vi "Subvi AO LUT mon.vi"(1 "AO mon":refnum<k21>="Connector1/AO1", 2 "AO":refnum<k21>="Connector1/AO0", 7 "Ext trig enable":bool, 9 "FIFO In":refnum<k21>="GALVO1mem") -> ()   [LabVIEW 2017]
uses:
  <vilib>/Platform/TimedLoop/XDataNode/timing_clust.ctl
  <vilib>/Platform/TimedLoop/XDataNode/nitl_modes.ctl
  <vilib>/Platform/TimedLoop/XDataNode/wakeup.ctl
  <vilib>/rvi/Emulation/niFpgaSctlEmulationGetInTimedLoop.vi
  <vilib>/rvi/Emulation/niFpgaEmulationReportErrorSimple.vi
  <vilib>/rvi/Emulation/niFpgaGetClockAttributes.vi
  <vilib>/rvi/Emulation/niFpgaCriticalErrorInLSC.vi
  Detector/GV gated frameclock.vi
  Detector/GV framegate.vi
  <vilib>/rvi/DataTransferAndStorage/Container/Common/niFpgaContainerExecOnDevCompGetState.vi
  <vilib>/rvi/Emulation/niFpgaEmulationIsFPGAContextNoSignature.vi
  <vilib>/rvi/DataTransferAndStorage/Container/Common/niFpgaContainerGetUniqueNameForEmu.vi
  <vilib>/rvi/Emulation/niFpgaProcessEmulError.vi
  <vilib>/rvi/errors/nirviReportUnexpectedCaseInternalError (U32).vi
  <vilib>/rvi/Memory/Memory_Emulation/niFpgaMemoryEmulationCacheClearOnFirstRun.vi
  <vilib>/rvi/Memory/Memory_Emulation/nirvimemoryEmulationManagerCache_MakeExclusive.vi
  <vilib>/rvi/Memory/Memory_Emulation/niFpgaMemoryEmulationValidateCache.vi
  <vilib>/rvi/Memory/Memory_Emulation/nirvimemoryEmulationManagerCache_InsertValue.vi
  <vilib>/Utility/error.llb/Clear Errors.vi
  <vilib>/rvi/Memory/Memory_Emulation/nirvimemoryEmulationManagerCache_ReleaseExclusive.vi
  <vilib>/rvi/Memory/Memory_Emulation/nirvimemoryEmulationManagerCache_GetValue.vi
  <vilib>/rvi/Memory/Memory_Emulation/nirvimemoryEmulationManagerCache_SetValue.vi
  <vilib>/rvi/Emulation/niFpgaSctlEmulationResourceMgr.vi
  <vilib>/rvi/eio/common/nirviEmuTemplateMethod_errors.vi
  <vilib>/Platform/TimedLoop/XDataNode/XDataNode.xnode
  <vilib>/rvi/DataTransferAndStorage/Container/XNode/niFpgaContainer.xnode
  <vilib>/rvi/Memory/Memory_Emulation/niFpgaMemoryEmulationRefIn.vi
  <vilib>/eio/EIONode/EIONode.xnode
  <vilib>/Platform/TimedLoop/XDataNode/XDNodeRunTimeDep.lvlib
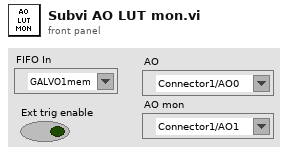
[diagram p1: front panel]
types:
  T1 = typedef "XDNodeRunTimeDep.lvlib/timing_clust.ctl" = cluster{"Expected End [f-1]":u64, "Actual End [f-1]":u64, "Finished Late? [f-1]":bool, "Expected End [i-1]":u64, "Actual End [i-1]":u64, "Finished Late? [i-1]":bool, "Expected Start [i]":u64, "Actual Start [i]":u64, "Expected Start [f]":u64, "Actual Start [f]":u64, "Source Name":string, "Structure Name":string, "Period":i64, "Deadline":i64, "Offset":i64, "Start":i64, "Priority":i32, "Timeout":i32, "Mode":T2, "Wakeup Reason":T3, "Error":errorcluster, "Source Type":string, "Secondary Source Type":string, "Global End Time":u64, "Global Start Time":u64, "Frame Duration":u64, "Iteration Duration":u64, "Assigned CPU":i32, "I/O Scan Engine Mode":u32}
  T2 = typedef "XDNodeRunTimeDep.lvlib/nitl_modes.ctl" = enum32{"No Change", "Process missed periods, maintain original phase", "Discard missed periods, maintain original phase", "Process missed periods, ignore original phase", "Discard missed periods, ignore original phase"}
  T3 = typedef "XDNodeRunTimeDep.lvlib/wakeup.ctl" = enum32{"Normal", "Aborted", "Asynchronous wakeup", "Timing source error", "Timed loop error", "Timeout"}
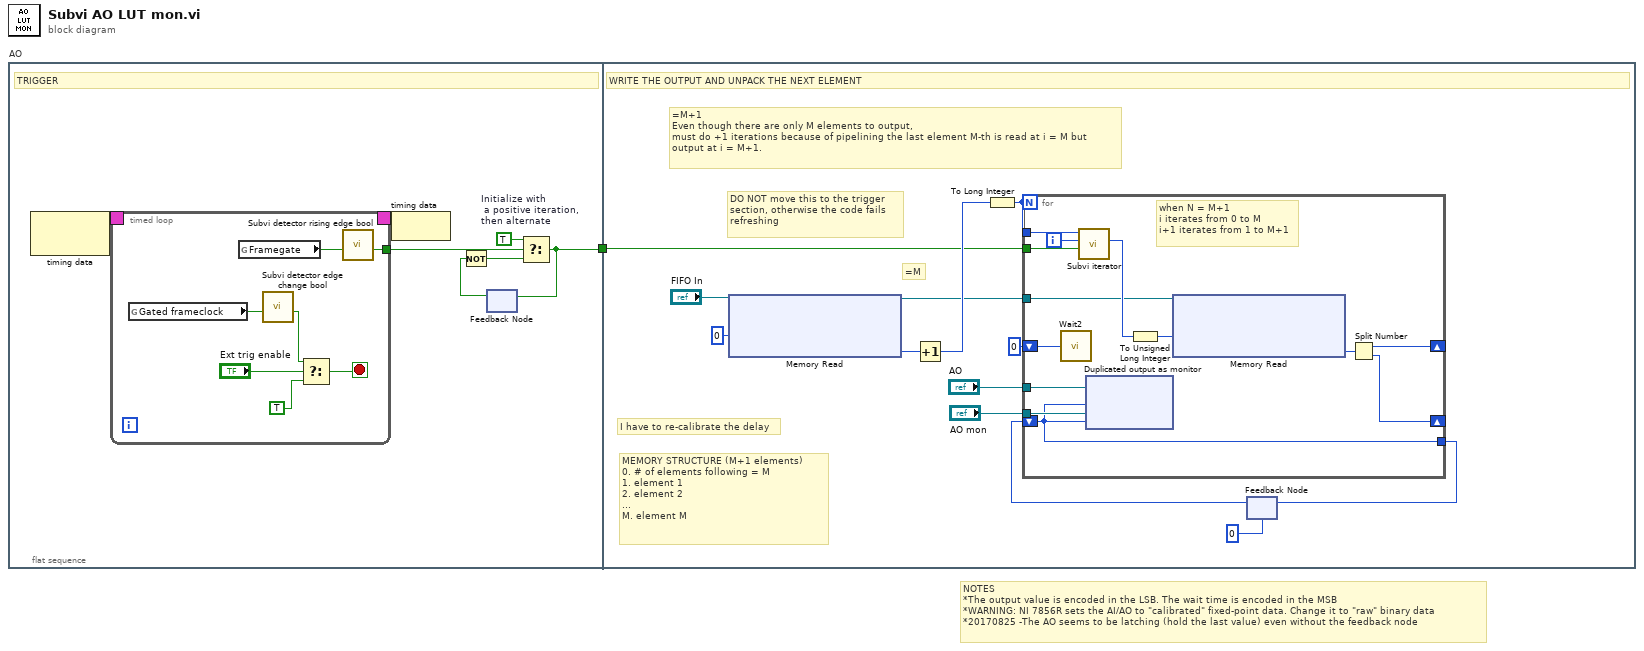
[diagram p0: block diagram]
diagram:
  # "NOTES\n*The output value is encoded in the LSB. The wait time is encoded in the MSB\n*WARNING: NI 7856R sets the AI/AO to \"calibrated\" fixed-point data. Change it to \"raw\" binary data\n*20170825 -The AO seems to be latching (hold the last value) even without the feedback node"
  n1 = flat-sequence "AO" {
    tunnel: [w2] -> w1
    tunnel: w1 -> [w24]
    frame #0 {
      # "TRIGGER"
      n2 = node-c288() -> (w8:T1)  [unwired: 1 in]
      n3 = timed-loop {
        timing: w8 -> [_]
        timing-out: [_] -> w7
        tunnel: [w9] -> w3
        stop <- w13 stop-if-true
        n4 = global read "GV gated frameclock.vi" "Gated frameclock"() -> (w12:bool)
        n5 = global read "GV framegate.vi" "Framegate"() -> (w10:bool)
        n6 = call "Subvi detector edge change bool.vi"("Input"=w12) -> ("Output"=w11:bool)  [unwired: 8 in]
        n7 = Select(t=w11, s="Ext trig enable", f=TRUE) -> (s? t:f=w13:bool)
        n8 = call "Subvi detector rising edge bool.vi"("Input"=w10) -> ("Output"=w9:bool)  [unwired: 10 in]
      }
      n9 = node-c288(w7) -> ()
      n10 = feedback #1() -> (w5:bool)  [unwired: 1 in]
      n11 = Not(x=w5) -> (.not. x?=w6:bool)
      n12 = Select "Initialize with\n a positive iteration,\nthen alternate"(t=TRUE, s=w3, f=w6) -> (s? t:f=w2:bool)
      n13 = feedback-in #1(w2) -> ()
    }
    frame #1 {
      # "DO NOT move this to the trigger\nsection, otherwise the code fails\nrefreshing"
      # "I have to re-calibrate the delay"
      # "MEMORY STRUCTURE (M+1 elements)\n0. # of elements following = M\n1. element 1\n2. element 2\n...\nM. element M"
      # "=M+1\nEven though there are only M elements to output,\nmust do +1 iterations because of pipelining the last element M-th is read at i = M but\noutput at i = M+1."
      # "=M"
      # "WRITE THE OUTPUT AND UNPACK THE NEXT ELEMENT"
      n14 = xnode ("Memory Read")("Address"=u32 0, "Memory In"="FIFO In") -> ("Data"=w26:u32, "Memory Out"=w25:refnum<k21>)
      n15 = Increment(x=w26) -> (x+1=w29:u32)
      n16 = To Long Integer(number=w29) -> (32bit integer=w28:i32)
      n17 = feedback #2(u16 0) -> (w32:u16)
      n18 = for {
        N: w28 -> [_]
        shift-right: [w43] -> _
        shift-left: u16 0 -> [w41]
        shift-right: [w42] -> _
        shift-left: w32 -> [w33]
        tunnel: [w33] -> w30
        tunnel: w28 -> [w38]
        tunnel: w24 -> [w37]
        tunnel: w25 -> [w36]
        tunnel: "AO mon" -> [w35]
        tunnel: "AO" -> [w34]
        i -> [w39]
        # "when N = M+1\ni iterates from 0 to M\ni+1 iterates from 1 to M+1"
        n19 = call "Wait2"("Count(Ticks)"=w41) -> ()  [unwired: 1 out]
        n20 = call "Subvi iterator.vi"("Set increase"=w37, "Iterator in"=w39, "Nmax"=w38) -> ("Iterator out"=w40:i32)  [unwired: 7 in, 1 out]
        n21 = xnode "Duplicated output as monitor"("I/O Item"=w33, "FPGA I/O In"=w34, "I/O Item"=w33, "FPGA I/O In"=w35) -> ()  [unwired: 2 out]
        n22 = To Unsigned Long Integer(number=w40) -> (unsigned 32bit integer=w45:u32)
        n23 = xnode ("Memory Read")("Address"=w45, "Memory In"=w36) -> ("Data"=w44:u32)  [unwired: 1 out]
        n24 = Split Number(x=w44) -> (hi(x)=w43:u16, lo(x)=w42:u16)
      }
      n25 = feedback-in #2(w30) -> ()
    }
  }
